vi "Read Histogram Hits.vi"(0 "VISA resource name":refnum<visa-resource-name>, 11 "error in (no error)":errorcluster) -> (3 "Histogram Total Hits":i32, 4 "VISA resource name out":refnum<visa-resource-name>, 6 "Histogram Hits in 3 Std Dev":dbl, 8 "Histogram Hits in 2 Std Dev":dbl, 10 "Histogram Hits in 1 Std Dev":dbl, 14 "Histogram Standard Deviation":dbl, 15 "error out":errorcluster)   [LabVIEW 2015, in "Agilent 2000 3000 X-Series.lvlib"]
doc: "Returns statistics related to histogram hit counts.\n\n<b>Note:</b>\nThis VI is specific to the 6000-X Series oscilloscopes. These features are not available on other models."
uses:
  <instrlib>/Agilent 2000 3000 X-Series/Agilent 2000 3000 X-Series.lvlib
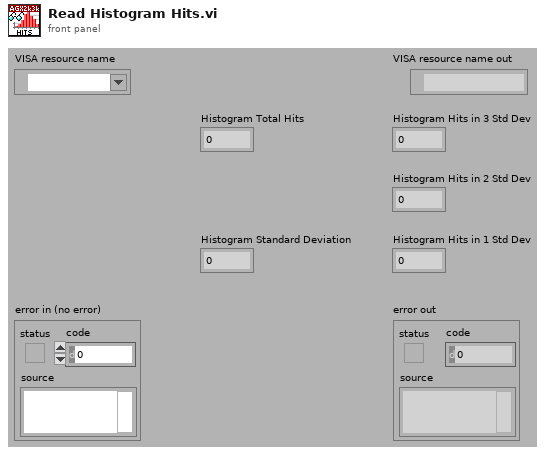
[diagram p1: front panel]
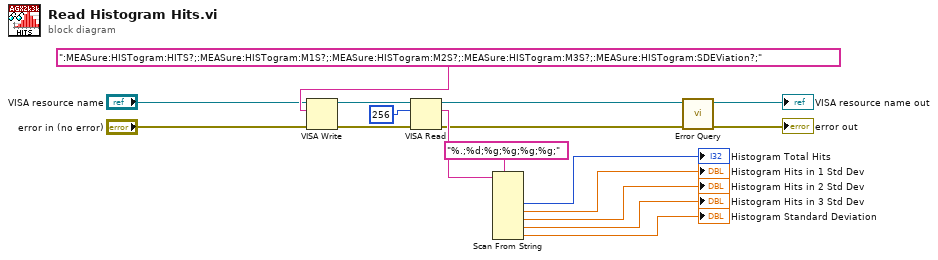
[diagram p0: block diagram]
diagram:
  n1 = VISA Write(VISA resource name="VISA resource name", write buffer=":MEASure:HISTogram:HITS?;:MEASure:HISTogram:M1S?;:MEASure:HISTogram:M2S?;:MEASure:HISTogram:M3S?;:MEASure:HISTogram:SDEViation?;", error in (no error)="error in (no error)") -> (VISA resource name out=w11:refnum<visa-resource-name>, error out=w10:errorcluster)  [unwired: 1 out]
  n2 = VISA Read(VISA resource name=w11, byte count=u32 256, error in (no error)=w10) -> (VISA resource name out=w4:refnum<visa-resource-name>, read buffer=w14:string, error out=w3:errorcluster)  [unwired: 1 out]
  n3 = Scan From String(format string="%.;%d;%g;%g;%g;%g;", input string=w14) -> (output 1=→"Histogram Total Hits":i32, output 2=→"Histogram Hits in 1 Std Dev":dbl, output 3=→"Histogram Hits in 2 Std Dev":dbl, output 4=→"Histogram Hits in 3 Std Dev":dbl, output 5=→"Histogram Standard Deviation":dbl)  [unwired: 7 in, 3 out]
  n4 = call <instrlib>:"Error Query.vi"("error in (no error)"=w3, "VISA resource name"=w4) -> ("error out"=→"error out":errorcluster, "VISA resource name out"=→"VISA resource name out":refnum<visa-resource-name>)  [unwired: 6 in, 2 out]
